vi "Get changed channel.vi"(9 "NewVal":T1, 10 "OldVal":T1, 11 "Cluster reference":refnum<vi>) -> (1 "Changed value":dbl, 2 "Changed channel":u8)   [LabVIEW 2016]
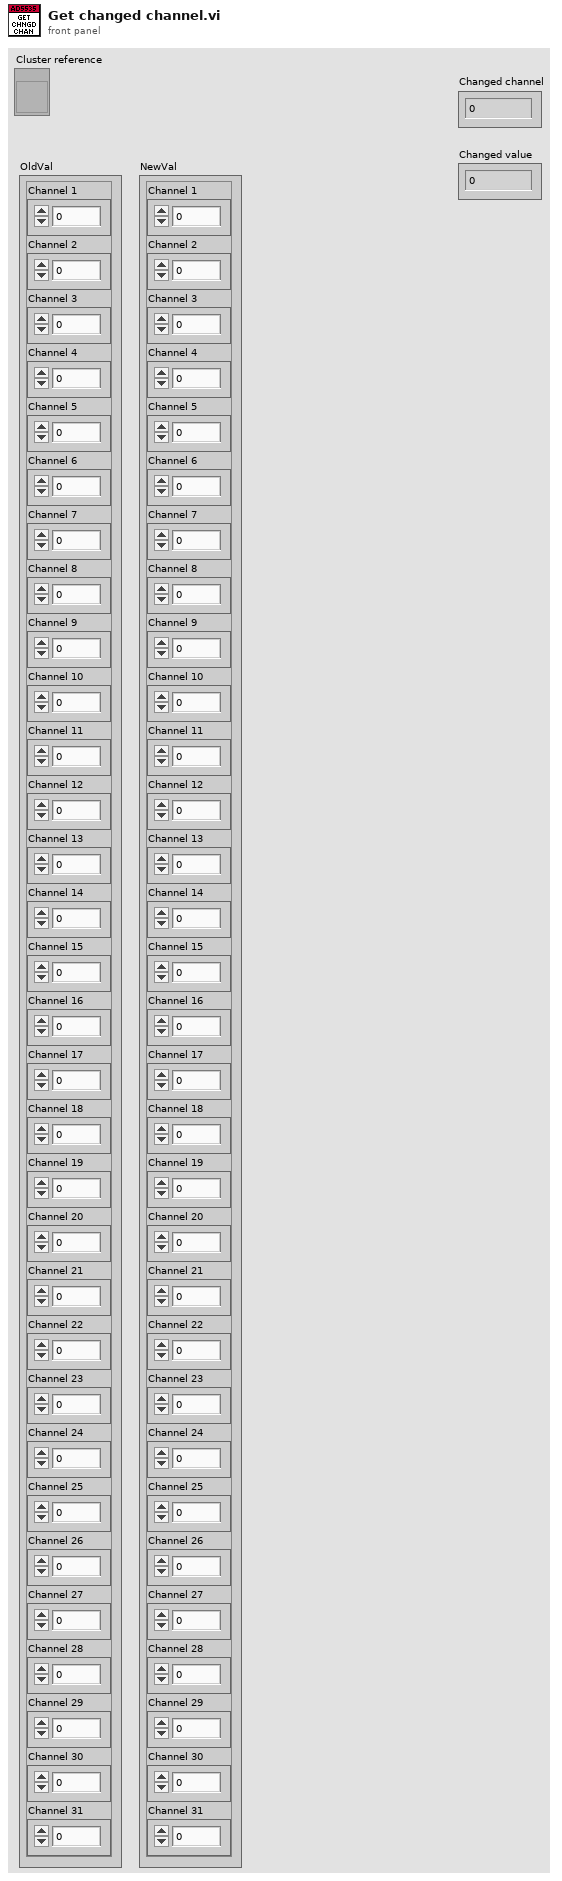
[diagram p1: front panel]
types:
  T1 = cluster{"Channel 1":dbl, "Channel 2":dbl, "Channel 3":dbl, "Channel 4":dbl, "Channel 5":dbl, "Channel 6":dbl, "Channel 7":dbl, "Channel 8":dbl, "Channel 9":dbl, "Channel 10":dbl, "Channel 11":dbl, "Channel 12":dbl, "Channel 13":dbl, "Channel 14":dbl, "Channel 15":dbl, "Channel 16":dbl, "Channel 17":dbl, "Channel 18":dbl, "Channel 19":dbl, "Channel 20":dbl, "Channel 21":dbl, "Channel 22":dbl, "Channel 23":dbl, "Channel 24":dbl, "Channel 25":dbl, "Channel 26":dbl, "Channel 27":dbl, "Channel 28":dbl, "Channel 29":dbl, "Channel 30":dbl, "Channel 31":dbl}
  T2 = cluster{"Channel 1":bool, "Channel 2":bool, "Channel 3":bool, "Channel 4":bool, "Channel 5":bool, "Channel 6":bool, "Channel 7":bool, "Channel 8":bool, "Channel 9":bool, "Channel 10":bool, "Channel 11":bool, "Channel 12":bool, "Channel 13":bool, "Channel 14":bool, "Channel 15":bool, "Channel 16":bool, "Channel 17":bool, "Channel 18":bool, "Channel 19":bool, "Channel 20":bool, "Channel 21":bool, "Channel 22":bool, "Channel 23":bool, "Channel 24":bool, "Channel 25":bool, "Channel 26":bool, "Channel 27":bool, "Channel 28":bool, "Channel 29":bool, "Channel 30":bool, "Channel 31":bool}
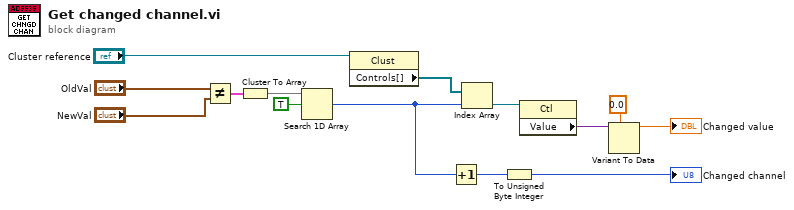
[diagram p0: block diagram]
diagram:
  n1 = Not Equal?(x="OldVal", y="NewVal") -> (x != y?=w14:T2)
  n2 = Cluster To Array(cluster=w14) -> (array=w12:bool[])
  n3 = Search 1D Array(1D array=w12, element=TRUE ("Element Data")) -> (index of element=w2:i32)  [unwired: 1 in]
  n4 = property class="Clust"(reference="Cluster reference") -> ("Controls[]"=w13:refnum<vi>[])  [unwired: 1 in, 2 out]
  n5 = Increment(x=w2) -> (x+1=w1:i32)
  n6 = Index Array(array=w13, index=w2) -> (element=w10:refnum<vi>)
  n7 = To Unsigned Byte Integer(number=w1) -> (unsigned 8bit integer=→"Changed channel":u8)
  n8 = property class="Ctl"(reference=w10) -> ("Value"=w9:variant)  [unwired: 1 in, 2 out]
  n9 = Variant To Data(type=0.0 ("Channel 1"), Variant=w9) -> (data=→"Changed value":dbl)  [unwired: 1 in, 1 out]
